vi "AutoNamerDatExtraArtem.vi"(3 "SweepType":string, 4 "ExtraString":string, 5 "Custom User Path":path) -> (0 "String":string, 2 "Path":path)   [LabVIEW 2021]
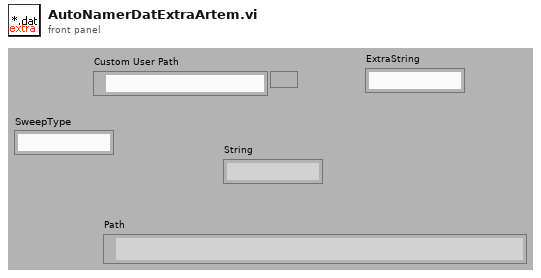
[diagram p1: front panel]
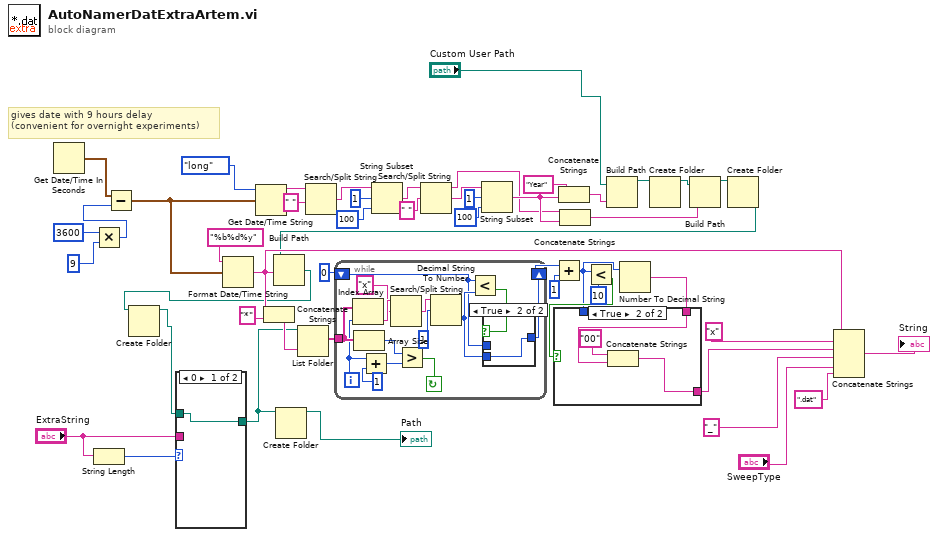
[diagram p0: block diagram]
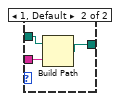
[diagram p2: hidden frame]
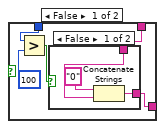
[diagram p4: hidden frame]
diagram:
  # "gives date with 9 hours delay\n(convenient for overnight experiments)"
  n1 = Get Date/Time In Seconds() -> (seconds since 1Jan1904=w10:timestamp)
  n2 = Multiply(x=3600, y=9) -> (x*y=w7:i32)
  n3 = String Length(string="ExtraString") -> (length=w6:i32)
  n4 = Subtract(x=w10, y=w7) -> (x-y=w4:timestamp)
  n5 = Format Date/Time String(time format string (%c)="%b%d%y", seconds (now)=w4) -> (date/time string=w21:string)  [unwired: 1 in]
  n6 = Get Date/Time String(date format (0)=enum16{"short", "long", "abbreviated"}."long", seconds (now)=w4) -> (date string=w36:string)  [unwired: 1 in, 1 out]
  n7 = Concatenate Strings(w21, "*") -> (w44:string)
  n8 = Search/Split String(string=w36, search string/char (-)=" ") -> (match + rest of string=w34:string)  [unwired: 1 in, 2 out]
  n9 = String Subset(string=w34, offset (0)=1, length (rest)=100 ("length (rest)")) -> (substring=w27:string)
  n10 = Search/Split String(string=w27, search string/char (-)=" ") -> (substring before match=w23:string, match + rest of string=w28:string)  [unwired: 1 in, 1 out]
  n11 = String Subset(string=w28, offset (0)=1, length (rest)=100 ("length (rest)")) -> (substring=w24:string)
  n12 = Concatenate Strings("Year" ("Substring"), w24) -> (w25:string)
  n13 = Concatenate Strings(w23, w24) -> (w22:string)
  n14 = Build Path(base path="Custom User Path", name or relative path=w25) -> (appended path=w20:path)
  n15 = Create Folder(path (use dialog)=w20) -> (created path=w19:path)  [unwired: 2 in, 2 out]
  n16 = Build Path(base path=w19, name or relative path=w22) -> (appended path=w18:path)
  n17 = Create Folder(path (use dialog)=w18) -> (created path=w17:path)  [unwired: 2 in, 2 out]
  n18 = Build Path(base path=w17, name or relative path=w21) -> (appended path=w11:path)
  n19 = Create Folder(path (use dialog)=w11) -> (created path=w12:path)  [unwired: 2 in, 2 out]
  n20 = case shown="0" w6 {
    tunnel: [w51 w54] -> w13
    tunnel: w12 -> [w51 w53]
    tunnel: "ExtraString" -> [_ w52]
    frame 0 {
    }
    frame 1, Default {
      n21 = Build Path(base path=w53, name or relative path=w52) -> (appended path=w54:path)
    }
  }
  n22 = Create Folder(path (use dialog)=w13) -> (created path=→"Path":path)  [unwired: 2 in, 2 out]
  n23 = List Folder(path=w13, pattern=w44) -> (filenames=w45:string[])  [unwired: 2 in, 3 out]
  n24 = while {
    shift-left: 0 -> [w61]
    shift-right: [w60] -> w47
    tunnel: w45 -> [w57]
    i -> [w56]
    stop <- w66 continue-if-true
    n25 = Index Array(array=w57, index=w56) -> (element=w65:string)
    n26 = Array Size(array=w57) -> (size(s)=w68:i32)
    n27 = Add(x=w56, y=1) -> (x+y=w55:i32)
    n28 = Search/Split String(string=w65, search string/char (-)="x") -> (match + rest of string=w59:string)  [unwired: 1 in, 2 out]
    n29 = Greater?(x=w68, y=w55) -> (0:w66:bool)
    n30 = Decimal String To Number(string=w59, offset=1) -> (number=w62:i32)  [unwired: 1 in, 1 out]
    n31 = Less?(x=w61, y=w62) -> (x < y?=w63:bool)
    n32 = case shown="True" w63 {
      tunnel: w62 -> [_ w70]
      tunnel: w61 -> [w69 _]
      tunnel: [w69 w70] -> w60
      frame False {
      }
      frame True {
      }
    }
  }
  n33 = Add(x=w47, y=1) -> (x+y=w39:i32)
  n34 = Less?(x=w39, y=10) -> (x < y?=w41:bool)
  n35 = Number To Decimal String(number=w39) -> (decimal integer string=w40:string)  [unwired: 1 in]
  n36 = case shown="True" w41 {
    tunnel: w40 -> [w72 w82]
    tunnel: [w71 w80] -> w38
    tunnel: w39 -> [w74 _]
    frame False {
      n37 = Greater?(x=w74, y=100) -> (0:w73:bool)
      n38 = case shown="False" w73 {
        tunnel: w72 -> [w77 w79]
        tunnel: [w76 w79] -> w71
        frame False {
          n39 = Concatenate Strings("0", w77) -> (w76:string)
        }
        frame True {
        }
      }
    }
    frame True {
      n40 = Concatenate Strings("00", w82) -> (w80:string)
    }
  }
  n41 = Concatenate Strings(w21, "x", w38, "_" ("string"), "SweepType", ".dat" ("Substring")) -> (→"String":string)
